vi "tofromrepo.vi"() -> ()   [LabVIEW 2013, in "async tests.lvlib"]
uses:
  async tests.lvlib
  Framework Configuration Classes/class cache/class metadata.ctl
  Framework Configuration Classes/class cache/PL_class cache.lvlib
  Framework Configuration Classes/class cache/cache definition.ctl
  <vilib>/NI/Tag Bus Module Framework/root configuration/TBM configuration.lvclass
  configuration/asynchronous execution module configuration.lvclass
  <vilib>/NI/Tag Bus Module Framework/module configuration/TBM module configuration.lvclass
  <vilib>/NI/Module Execution Interface/Engine Configuration/engine configuration.lvclass
  Framework Configuration Classes/platypus configuration/engines cluster.ctl
  Framework Configuration Classes/platypus configuration/PLConfigurationSerializer.lvlib
  Configuration Editor/Classes/SystemConfigRepo/SystemConfigRepo.lvclass
  Configuration Editor/Classes/Asynchronous Component Editor Node/Asynchronous Module Editor Node.lvclass
  <vilib>/CEF_TreeControl/Node/FromRepoCluster.ctl
  <vilib>/CEF_TreeControl/Node/NISE_CEF_Node.lvclass
  Configuration Editor/Classes/Module editor node/to repo data.ctl
  Configuration Editor/Classes/Module editor node/module editor node.lvclass
  <vilib>/CEF_TreeControl/Node/ToRepoCluster.ctl
  Framework Configuration Classes/system configuration/PL_System Configuration.lvclass
  Framework Configuration Classes/target configuration/PL_Target Configuration.lvclass
  Framework Configuration Classes/platypus configuration/targets cluster.ctl
  Framework Configuration Classes/platypus configuration/systems cluster.ctl
  tests/test module/module/configuration/TEST CONFIGURATION.lvclass
  tests/test module/editor node/TEST EDITOR.lvclass
  Configuration Editor/Classes/TBM Configuration Node/TBM Configuration Node.lvclass
  Framework Configuration Classes/class cache/cached class information.ctl
  Framework Configuration Classes/class cache/cache search configuration.ctl
panel:
  out "repo cfg ok":bool
  out "editor cfg ok":bool
  out "async t/o ok":bool
  out "async ok?":bool
  out "no error lol":errorcluster
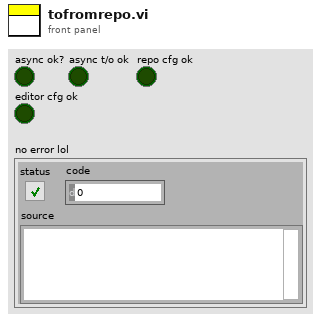
[diagram p1: front panel]
types:
  T1 = typedef "PL_class cache.lvlib/cache definition.ctl" = cluster{"configuration":T2, "class cache data":T3}
  T2 = typedef "PL_class cache.lvlib/cache search configuration.ctl" = cluster{"Search Paths":path[], "Folders to Exclude":string[], "full class list":path[]}
  T3 = typedef "PL_class cache.lvlib/cached class information.ctl" = cluster{"targets":T4[], "engines":T4[], "modules":T4[], "ignored class list":path[]}
  T4 = typedef "PL_class cache.lvlib/class metadata.ctl" = cluster{"file name":string, "fully qualified name":string, "menu display name":string, "configuration class":string, "instances allowed":i32}
  T5 = typedef "PLConfigurationSerializer.lvlib/targets cluster.ctl" = cluster{"Target Configuration":refnum<class "PL_Target Configuration.lvclass">, "engines":T6[]}
  T6 = typedef "PLConfigurationSerializer.lvlib/engines cluster.ctl" = cluster{"engine configuration":refnum<class "engine configuration.lvclass">, "modules":refnum<class "TBM module configuration.lvclass">[]}
  T7 = typedef "PLConfigurationSerializer.lvlib/systems cluster.ctl" = cluster{"System Configuration":refnum<class "PL_System Configuration.lvclass">, "targets":T5[]}
  T8 = typedef "PL Framework Configuration Tool.lvlib/module editor node.lvclass/to repo data.ctl" = cluster{"target index":i32, "engine index":i32}
  T9 = typedef "NISE_CEF_Node.lvclass/FromRepoCluster.ctl" = cluster{"tag":string, "tags":string[], "classes":string[], "index":i32, "variant":variant}
  T10 = typedef "NISE_CEF_Node.lvclass/ToRepoCluster.ctl" = cluster{"variant":variant}
  T11 = typedef "NISE_CEF_Node.lvclass/NodeRef.ctl" = refnum<data-value>
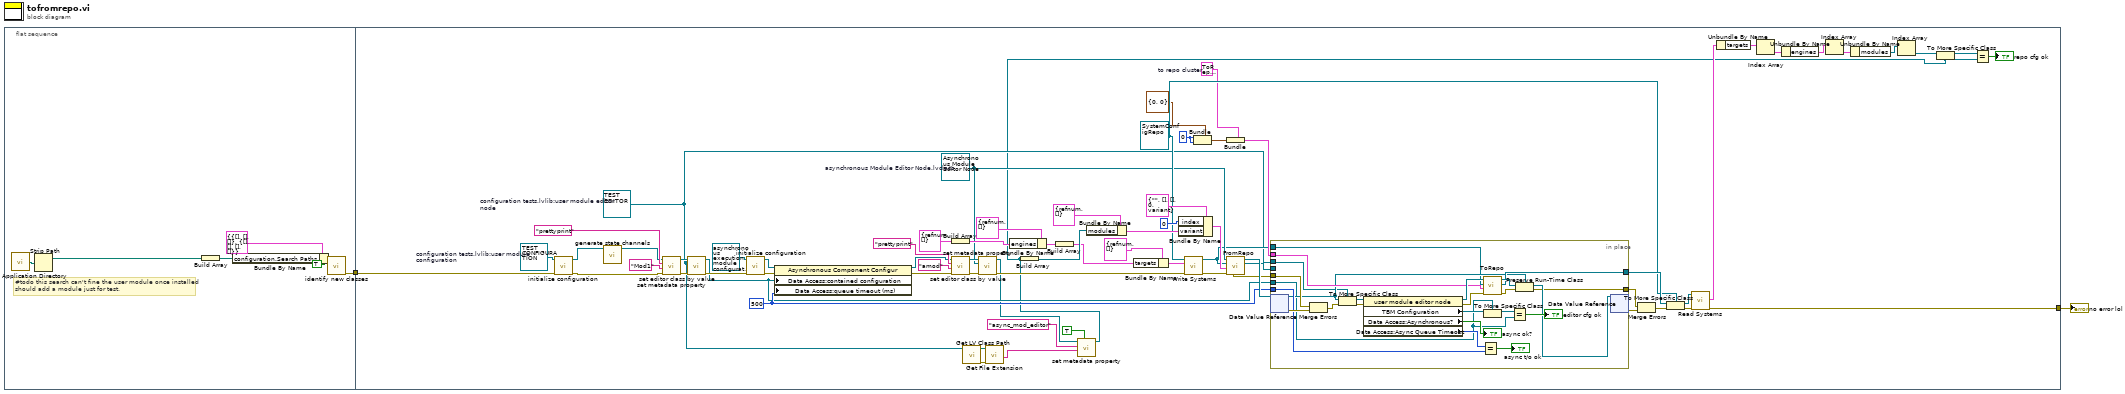
[diagram p0: block diagram]
diagram:
  n1 = flat-sequence {
    tunnel: [w7] -> w1
    tunnel: [w59] -> w2
    tunnel: w1 -> [w34]
    frame #0 {
      # "#todo this search can't fine the user module once installed\nshould add a module just for test."
      n2 = call <vilib>:"Application Directory.vi"() -> ("Application Directory"=w3:path)
      n3 = Strip Path(path=w3) -> (stripped path=w4:path)  [unwired: 1 out]
      n4 = Build Array(w4) -> (w5:path[])
      n5 = Bundle By Name(cluster=T1 {"configuration"={"Search Paths"=[], "Folders to Exclude"=[], "full class list"=[]}, "class cache data"={"targets"=[], "engines"=[], "modules"=[], "ignored class list"=[]}} ("cache"), "configuration.Search Paths"=w5) -> (w9:T1)
      n6 = call "identify new classes.vi"("force scan"=TRUE, "cache in"=w9) -> ("error out"=w7:errorcluster)  [unwired: 8 in, 1 out]
    }
    frame #1 {
      w13 = refnum<class "TEST EDITOR.lvclass"> refnum  # configuration tests.lvlib:user module editor node
      w24 = refnum<class "TEST CONFIGURATION.lvclass"> refnum  # configuration tests.lvlib:user module configuration
      w51 = T10 {"variant"=variant}  # to repo cluster
      w52 = 0 ("target index")
      w25 = refnum<class "Asynchronous Module Editor Node.lvclass"> refnum  # asynchronous Module Editor Node.lvclass
      w54 = refnum<class "SystemConfigRepo.lvclass"> refnum ("PL Framework Configuration Tool.lvlib:SystemConfigRepo.lvclass")
      w62 = 500 ("queue timeout (ms)")
      n7 = call-dynamic "initialize configuration.vi"("error in"=w34, "configuration in"=w24) -> ("error out"=w21:errorcluster, "configuration out"=w23:refnum<class "TEST CONFIGURATION.lvclass">)  [unwired: 7 in, 1 out]
      n8 = call "generate state channels.vi"("tag bus configurable plugin module configuration in"=w23) -> ("tag bus configurable plugin module configuration out"=w22:refnum<class "TEST CONFIGURATION.lvclass">)  [unwired: 9 in, 1 out]
      n9 = call <vilib>:"set metadata property.vi"("error in"=w21, "value"="Mod1" ("format string"), "key"="prettyprint", "configuration in"=w22) -> ("error out"=w75:errorcluster, "configuration out"=w30:refnum<class "TEST CONFIGURATION.lvclass">)  [unwired: 6 in]
      n10 = call "set editor class by value.vi"("error in"=w75, "editor"=w13, "configuration in"=w30) -> ("error out"=w31:errorcluster, "configuration out"=w29:refnum<class "TEST CONFIGURATION.lvclass">)  [unwired: 7 in]
      n11 = call-dynamic "initialize configuration.vi"("error in"=w31, "configuration in"=refnum<class "asynchronous execution module configuration.lvclass"> refnum ("Asynchronous Component Configuration")) -> ("error out"=w76:errorcluster, "configuration out"=w77:refnum<class "asynchronous execution module configuration.lvclass">)  [unwired: 7 in, 1 out]
      n12 = property class="Asynchronous Component Configur"(reference=w77, error in=w76, "Data Access:contained configuration"=w29, "Data Access:queue timeout (ms)"=w62) -> (reference out=w72:refnum<class "asynchronous execution module configuration.lvclass">, error out=w71:errorcluster)
      n13 = Build Array(T6 {"engine configuration"=refnum, "modules"=[]} ("engines cluster")) -> (w45:T6[])
      n14 = call <vilib>:"set metadata property.vi"("error in"=w71, "value"="amod" ("format string"), "key"="prettyprint", "configuration in"=w72) -> ("error out"=w28:errorcluster, "configuration out"=w26:refnum<class "asynchronous execution module configuration.lvclass">)  [unwired: 6 in]
      n15 = call <vilib>:"Get LV Class Path.vi"("object"=w13) -> ("error out"=w15:errorcluster, "class path"=w16:path)  [unwired: 9 in]
      n16 = call "set editor class by value.vi"("error in"=w28, "editor"=w25, "configuration in"=w26) -> ("error out"=w27:errorcluster, "configuration out"=w11:refnum<class "asynchronous execution module configuration.lvclass">)  [unwired: 7 in]
      n17 = call <vilib>:"Get File Extension.vi"("error in (no error)"=w15, "file"=w16) -> ("filename without extension"=w14:string)  [unwired: 6 in, 3 out]
      n18 = Bundle By Name(cluster=T5 {"Target Configuration"=refnum, "engines"=[]} ("targets cluster"), "engines"=w45) -> (w46:T5)
      n19 = Build Array(w46) -> (w47:T5[])
      n20 = call <vilib>:"set metadata property.vi"("overwrite?"=TRUE, "value"=w14, "key"="async_mod_editor", "configuration in"=w11) -> ("configuration out"=w10:refnum<class "asynchronous execution module configuration.lvclass">)  [unwired: 6 in, 1 out]
      n21 = Build Array(w10) -> (w66:refnum<class "asynchronous execution module configuration.lvclass">[])
      n22 = Bundle By Name(cluster=T6 {"engine configuration"=refnum, "modules"=[]} ("engines cluster"), "modules"=w66) -> (w67:T6)
      n23 = Bundle By Name(cluster=T7 {"System Configuration"=refnum, "targets"=[]} ("system"), "targets"=w47) -> (w43:T7)
      n24 = Bundle By Name(cluster=T9 {"tag"="", "tags"=[], "classes"=[], "index"=0, "variant"=variant} ("from repo cluster"), "index"=0, "variant"=w67) -> (w65:T9)
      n25 = call "Write Systems.vi"("error in"=w27, "system"=w43, "SystemConfigRepo in"=w54) -> ("error out"=w55:errorcluster, "SystemConfigRepo out"=w18:refnum<class "SystemConfigRepo.lvclass">)  [unwired: 7 in]
      n26 = Bundle(cluster=T8 {"target index"=0, "engine index"=0} ("to repo data"), "target index"=w52, "engine index"=w52) -> (w49:T8)
      n27 = Bundle(cluster=w51, "variant"=w49) -> (w50:T10)
      n28 = call-dynamic "FromRepo.vi"("error in"=w55, "from repo cluster"=w65, "repository in"=w18, "Component in"=w25) -> ("error out"=w63:errorcluster, "repository out"=w61:refnum<class "NISE_CEF_Repository.lvclass">, "node"=w64:T11)  [unwired: 5 in]
      n29 = in-place {
        in-place-border: w63 -> [w104]
        in-place-border: [w85] -> w60
        in-place-border: w62 -> [w96]
        in-place-border: w29 -> [w82]
        in-place-border: w61 -> [_]
        in-place-border: [w90] -> w57
        in-place-border: w50 -> [w89]
        in-place-border: w13 -> [w84]
        in-place-border: w18 -> [w81]
        n30 = in-place-dvr #1(w64) -> (w87:refnum<class "NISE_CEF_Node.lvclass">, w103:errorcluster)
        n31 = Merge Errors(w104, w103) -> (w101:errorcluster)
        n32 = To More Specific Class(target class=w84, reference=w87, error in=w101) -> (specific class reference=w102:refnum<class "TEST EDITOR.lvclass">, error out=w100:errorcluster)
        n33 = property class="user module editor node"(reference=w102, error in=w100) -> (reference out=w93:refnum<class "TEST EDITOR.lvclass">, error out=w91:errorcluster, "TBM Configuration"=w95:refnum<class "TBM configuration.lvclass">, "Data Access:Asynchronous?"=→"async ok?":bool, "Data Access:Async Queue Timeout"=w98:i32)
        n34 = Equal?(x=w98, y=w96) -> (x = y?=→"async t/o ok":bool)
        n35 = call-dynamic "ToRepo.vi"("error in"=w91, "to repo cluster"=w89, "repository in"=w81, "node in"=w93) -> ("error out"=w86:errorcluster, "repository out"=w90:refnum<class "NISE_CEF_Repository.lvclass">, "node out"=w92:refnum<class "TEST EDITOR.lvclass">)  [unwired: 5 in]
        n36 = To More Specific Class(target class=w82, reference=w95) -> (specific class reference=w83:refnum<class "TEST CONFIGURATION.lvclass">)  [unwired: 1 in, 1 out]
        n37 = Equal?(x=w83, y=w82) -> (x = y?=→"editor cfg ok":bool)
        n38 = Preserve Run-Time Class(object in=w92, error in=w86, 2:w87) -> (object out=w88:refnum<class "NISE_CEF_Node.lvclass">, error out=w85:errorcluster)
        n39 = in-place-dvr #1(w88) -> (w32:errorcluster)  [unwired: 1 out]
      }
      n40 = Merge Errors(w60, w32) -> (w33:errorcluster)
      n41 = To More Specific Class(target class=w54, reference=w57, error in=w33) -> (specific class reference=w56:refnum<class "SystemConfigRepo.lvclass">, error out=w58:errorcluster)
      n42 = call "Read Systems.vi"("error in"=w58, "SystemConfigRepo in"=w56) -> ("error out"=w59:errorcluster, "system"=w41:T7)  [unwired: 7 in, 1 out]
      n43 = Unbundle By Name(w41) -> ("targets"=w40:T5[])
      n44 = Index Array(array=w40) -> (element=w38:T5)  [unwired: 1 in]
      n45 = Unbundle By Name(w38) -> ("engines"=w39:T6[])
      n46 = Index Array(array=w39) -> (element=w36:T6)  [unwired: 1 in]
      n47 = Unbundle By Name(w36) -> ("modules"=w37:refnum<class "TBM module configuration.lvclass">[])
      n48 = Index Array(array=w37) -> (element=w35:refnum<class "TBM module configuration.lvclass">)  [unwired: 1 in]
      n49 = To More Specific Class(target class=w10, reference=w35) -> (specific class reference=w20:refnum<class "asynchronous execution module configuration.lvclass">)  [unwired: 1 in, 1 out]
      n50 = Equal?(x=w20, y=w10) -> (x = y?=→"repo cfg ok":bool)
    }
  }
  "no error lol" <- w2
